vi "Table Caption.vi"(8 "error IN":errorcluster, 10 "Caption IN":string, 11 "PDF Report IN":T21(xcontrol)) -> (0 "error OUT":errorcluster, 1 "Caption position":enum16{"No caption", "Above", "Below"}(ring), 2 "Paragraph Refnum":refnum<k24>, 3 "PDF Report OUT":T21(xcontrol))   [LabVIEW 2013]
doc: "Version 1.0\nDeveloped by Jean-Marc Simard\nCopyright © 2010, Exaprom Inc.\nAll rights reserved.\nLicense: BSD\n\nWith iTextSharp 4.1.6 (http://itextsharp.sourceforge.net)\nunder Mozilla Public License Version 1.1\n(http://www.mozilla.org/MPL/MPL-1.1.html)"
uses:
  Controls/PDF Report Xcontrol/PDF Report.xctl
  C:/Users/MaxCorp/Documents/GitHub/TopView/DLL/itextsharp.dll
  DLL/itextsharp.dll
  Controls/Paragraphe cluster.ctl
  Controls/Texte alignement.ctl
  Controls/Line spacing.ctl
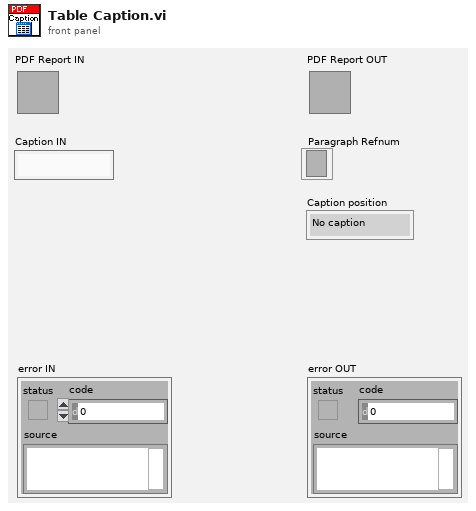
[diagram p1: front panel]
types:
  T1 = typedef "Font cluster.ctl" = cluster{"Name":string, "Size":T2, "Color":T3, "Style":cluster{"Bold":bool, "Italic":bool, "Underline":bool, "Strikeout":bool}}
  T2 = typedef "Font size.ctl" = sgl
  T3 = typedef "Font color.ctl" = u32
  T4 = typedef "Unit.ctl" = enum16{"inch", "mm"}
  T5 = typedef "Paragraphe cluster.ctl" = cluster{" Aligment":T6, "Line spacing":T7}
  T6 = typedef "Texte alignement.ctl" = enum16{"Select", "CENTER", "JUSTIFY", "LEFT", "RIGHT"}
  T7 = typedef "Line spacing.ctl" = enum16{"Select", "1.0", "1.5", "2.0"}
  T8 = typedef "Page dimensions.ctl" = cluster{"Start at page":i32, "Orientation":T9, "widht":sgl, "height":sgl, "Margin left":sgl, "Margin right":sgl, "Margin top":sgl, "Margin bottom":sgl}
  T9 = typedef "Page Orientation.ctl" = enum16{"Portrait", "Landscape"}
  T10 = typedef "Image or Table Caption.ctl" = cluster{"Caption":string, "Separator":string, "Position":enum16{"Above", "Below"}}
  T11 = typedef "Header Footer [ ].ctl" = T12[]
  T12 = typedef "Header Footer cluster.ctl" = cluster{"Start page":i32, "Type":T13, "Alignment":T14, "Vertical Alignement":T15, "Image (%)":sgl, "Page #":T16, "Text":string, "Path":string, "Font":T1, "Font refnum":refnum<k24>, "Line":cluster{"Line":T17, "Thickness (points)":sgl, "Colour":T3}}
  T13 = typedef "Header Footer Type.ctl" = enum16{"Select", "Text", "Text + hyperlink", "Page number", "Image", "Image + hyperlink"}
  T14 = typedef "Header footer horiz alignment.ctl" = enum16{"Left", "Center", "Right"}
  T15 = typedef "Cell Vertical alignment.ctl" = enum16{"TOP", "MIDDLE", "BOTTOM"}
  T16 = typedef "Page number.ctl" = cluster{"Text 1":string, "Text 2":string, "Text 3":string}
  T17 = typedef "Header Footer Line.ctl" = enum16{"No line", "Horizontal line"}
  T18 = typedef "Watermark cluster2.ctl" = cluster{"Show? (F)":bool, "Type":enum16{"Image", "Text"}, "Opacity (%)":sgl, "Rotate(°)":sgl, "Position":cluster{"Position":T19, "X":sgl, "Y":sgl}, "Image path":path, "Scaled(%)":sgl, "Image refnum":refnum<k24>, "Text":string, "Font":cluster{"Name":string, "Size":T2, "Color":T3}, "Font refnum":refnum<k24>, "Alignment":T14, "Automatic":bool}
  T19 = typedef "Watermark Position.ctl" = enum16{"Absolute", "Center (page)", "Center (text section)"}
  T20 = typedef "System Fonts.ctl" = cluster{"Font name [ ]":string[], "Font and file names [ ]":cluster{"Font name":string, "File name":string}[]}
  T21 = cluster{"Document":refnum<k24>, "Writer":refnum<k24>, "Default Font":refnum<k24>, "Default Font cluster":T1, "Path":path, "Unit (default = mm)":T4, "Paragraphe cluster":T5, "Pages dimensions [ ]":T8[], "Captions":cluster{"Image":T10, "Image counter":u16, "Table":T10, "Table counter":u16, "Font":T1}, "Header":T11, "Footer":T11, "Watermark ":T18, "Actual VI name":string, "System Fonts":T20}
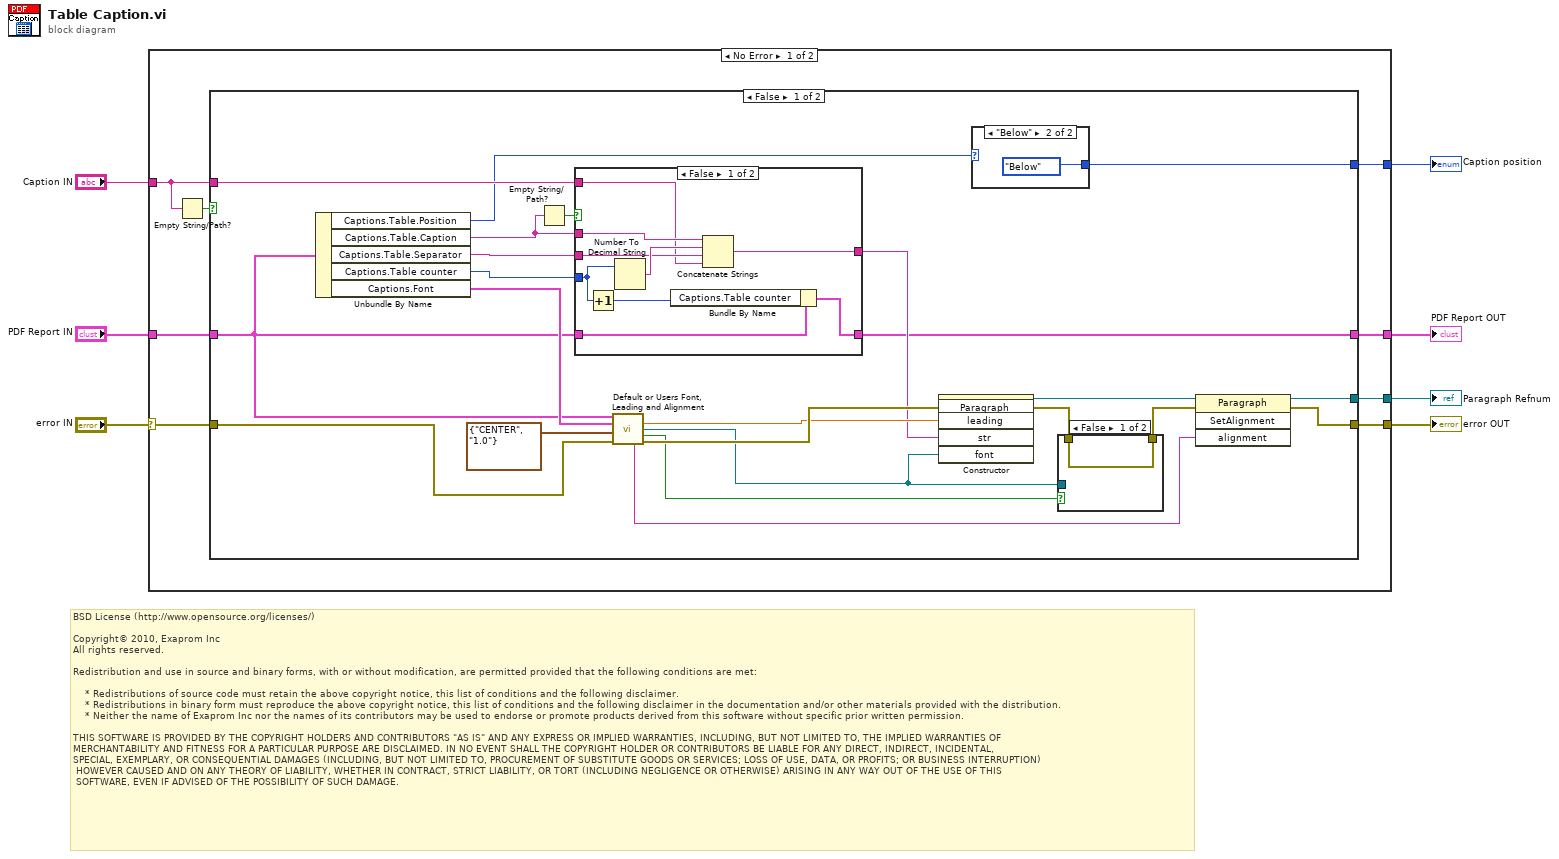
[diagram p0: block diagram]
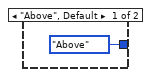
[diagram p2: hidden frame]
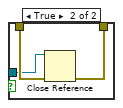
[diagram p3: hidden frame]
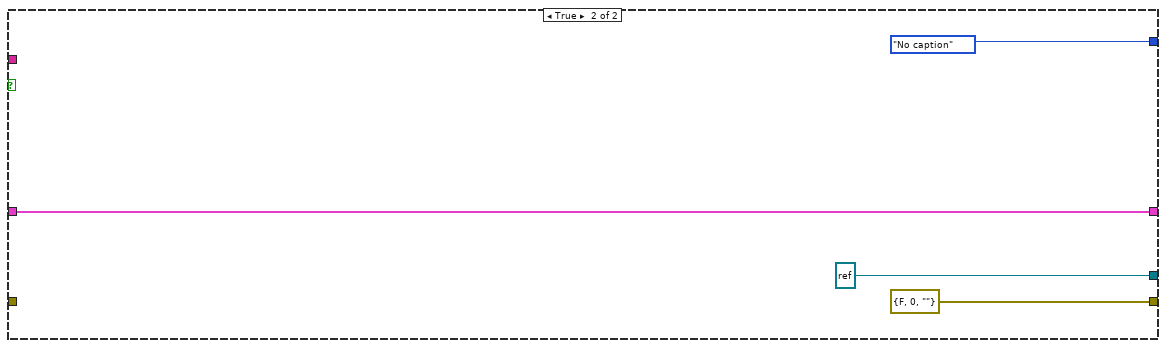
[diagram p5: hidden frame]
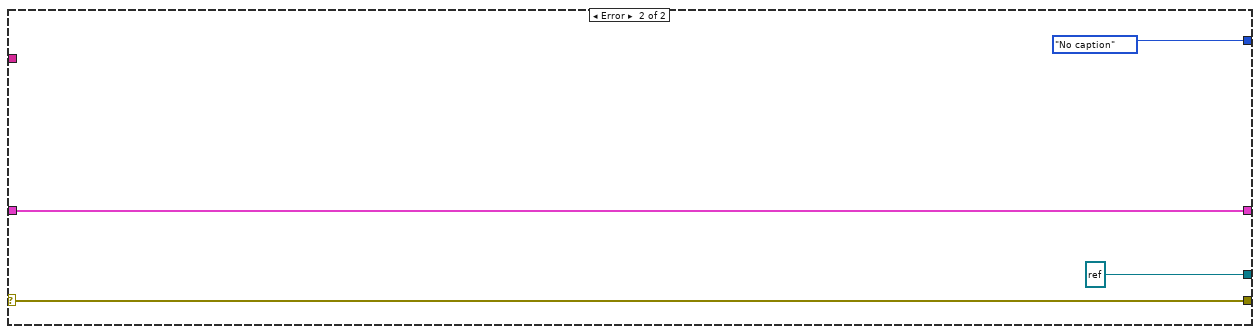
[diagram p6: hidden frame]
diagram:
  # "BSD License (http://www.opensource.org/licenses/)\n\nCopyright© 2010, Exaprom Inc\nAll rights reserved.\n\nRedistribution and use in source and binary forms, with or without modification, are permitted provided that the following conditions are met:\n\n    * Redistributions of source code must retain the above copyright notice, this list of conditions and the following disclaimer.\n    * Redistributions in binary form must reproduce the above copyright notice, this list of conditions and the following disclaimer in the documentation and/or other materials provided with the distribution.\n    * Neither the name of Exaprom Inc nor the names of its contributors may be used to endorse or promote products derived from this software without specific prior written permission.\n\nTHIS SOFTWARE IS PROVIDED BY THE COPYRIGHT HOLDERS AND CONTRIBUTORS \"AS IS\" AND ANY EXPRESS OR IMPLIED WARRANTIES, INCLUDING, BUT NOT LIMITED TO, THE IMPLIED WARRANTIES OF \nMERCHANTABILITY AND FITNESS FOR A PARTICULAR PURPOSE ARE DISCLAIMED. IN NO EVENT SHALL THE COPYRIGHT HOLDER OR CONTRIBUTORS BE LIABLE FOR ANY DIRECT, INDIRECT, INCIDENTAL,\nSPECIAL, EXEMPLARY, OR CONSEQUENTIAL DAMAGES (INCLUDING, BUT NOT LIMITED TO, PROCUREMENT OF SUBSTITUTE GOODS OR SERVICES; LOSS OF USE, DATA, OR PROFITS; OR BUSINESS INTERRUPTION)\n HOWEVER CAUSED AND ON ANY THEORY OF LIABILITY, WHETHER IN CONTRACT, STRICT LIABILITY, OR TORT (INCLUDING NEGLIGENCE OR OTHERWISE) ARISING IN ANY WAY OUT OF THE USE OF THIS\n SOFTWARE, EVEN IF ADVISED OF THE POSSIBILITY OF SUCH DAMAGE."
  n1 = case shown="No Error" "error IN" {
    selector: "error IN" -> [w8 w63]
    tunnel: [w15 w62] -> w7
    tunnel: "Caption IN" -> [w10 _]
    tunnel: "PDF Report IN" -> [w14 w62]
    tunnel: [w13 w63] -> w4
    tunnel: [w12 refnum<k24> refnum ("new reference")] -> w1
    tunnel: [w9 enum16{"No caption", "Above", "Below"}."No caption" ("Caption position")] -> w2
    frame No Error {
      n2 = Empty String/Path?(string/path=w10) -> (empty?=w11:bool)
      n3 = case shown="False" w11 {
        tunnel: [w20 w59] -> w15
        tunnel: w10 -> [w32 _]
        tunnel: w14 -> [w19 w59]
        tunnel: [w17 errorcluster {"status"=FALSE, "code"=0, "source"=""} ("error out")] -> w13
        tunnel: [w18 refnum<k24> refnum ("new reference")] -> w12
        tunnel: [w21 enum16{"No caption", "Above", "Below"}."No caption" ("Caption position")] -> w9
        tunnel: w8 -> [w16 _]
        frame False {
          n4 = Unbundle By Name(w19) -> ("Captions.Table.Position"=w22:enum16{"Above", "Below"}, "Captions.Table.Caption"=w33:string, "Captions.Table.Separator"=w34:string, "Captions.Table counter"=w35:u16, "Captions.Font"=w37:T1)
          n5 = Empty String/Path?(string/path=w33) -> (empty?=w31:bool)
          n6 = case shown="False" w31 {
            tunnel: w32 -> [w50 w55]
            tunnel: w33 -> [w53 _]
            tunnel: w34 -> [w51 _]
            tunnel: w35 -> [w49 _]
            tunnel: [w46 w55] -> w26
            tunnel: w19 -> [w48 w54]
            tunnel: [w45 w54] -> w20
            frame False {
              n7 = Increment(x=w49) -> (x+1=w47:u16)
              n8 = Number To Decimal String(number=w49) -> (decimal integer string=w52:string)  [unwired: 1 out]
              n9 = Bundle By Name(cluster=w48, "Captions.Table counter"=w47) -> (w45:T21)
              n10 = Concatenate Strings(w53, w52, w51, w50) -> (w46:string)
            }
            frame True {
            }
          }
          n11 = call "Default or Users Font, Leading and Alignment.vi"("PDF Report"=w19, "Font"=w37, "Paragraphe cluster"=T5 {" Aligment"=enum."CENTER", "Line spacing"=enum."1.0"}, "error in (no error)"=w16) -> ("Leading"=w30:T2, "Font Ref"=w29:refnum<k24>, "Close Font Ref"=w27:bool, "Aligment"=w28:string, "error out"=w38:errorcluster)  [unwired: 7 out]
          n12 = constructor class="Paragraph"(error in=w38, "leading"=w30, "str"=w26, "font"=w29) -> (reference out=w25:refnum<k24>, error out=w24:errorcluster)  [unwired: 2 in, 4 out]
          n13 = case shown="\"Below\"" w22 {
            tunnel: [enum16{"No caption", "Above", "Below"}."Above" ("Caption position") enum16{"No caption", "Above", "Below"}."Below" ("Caption position")] -> w21
            frame "Above", Default {
            }
            frame "Below" {
            }
          }
          n14 = case shown="False" w27 {
            tunnel: w24 -> [w41 w44]
            tunnel: [w41 w43] -> w23
            tunnel: w29 -> [_ w42]
            frame False {
            }
            frame True {
              n15 = Close Reference(reference=w42, error in (no error)=w44) -> (error out=w43:errorcluster)
            }
          }
          n16 = invoke class="Paragraph" method="SetAlignment"(reference=w25, error in=w23, "alignment"=w28) -> (reference out=w18:refnum<k24>, error out=w17:errorcluster)  [unwired: 1 in, 2 out]
        }
        frame True {
        }
      }
    }
    frame Error {
    }
  }
  "PDF Report OUT" <- w7
  "error OUT" <- w4
  "Caption position" <- w2
  "Paragraph Refnum" <- w1
